vi "Can Connect Channels.vi"(8 "error in (no error)":errorcluster, 9 "channel 2":string, 10 "channel 1":string, 11 "session in":T2) -> (0 "error out":errorcluster, 2 "path capability":T1=1 items=["Path Available"=1, "Path Exists"=2, "Path Unsupported"=3, "Resource in Use"=4, "Source Conflict"=5, "Channel Not Available"=6], 3 "session out":T2)   [LabVIEW 2020, in "SLSC Switch.lvlib"]
doc: "Verifies that a path between <B>channel 1</B> and <B>channel 2</B> can be created.\n\nIf a path is possible in the switch module, the availability of that path is returned given the existing connections. If the path is possible but in use, an Implicit Connection Exists warning is returned."
uses:
  <vilib>/SLSC_Switch/SLSC Switch.lvlib
  nislscsl.dll
  <vilib>/userdefined/High Color/SLSC_Switch/nislscslSession.ctl
  <vilib>/SLSC_Switch/Path Capability.ctl
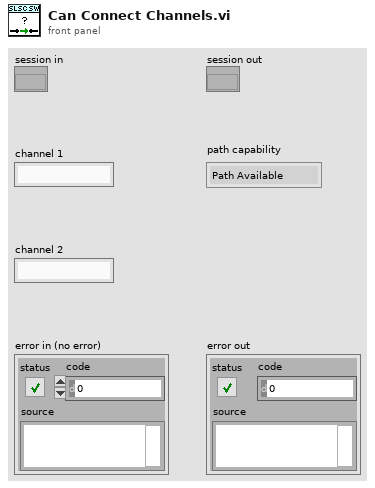
[diagram p1: front panel]
types:
  T1 = typedef "SLSC Switch.lvlib/Path Capability.ctl" = i32
  T2 = typedef "nislscslSession.ctl" = refnum<k20>
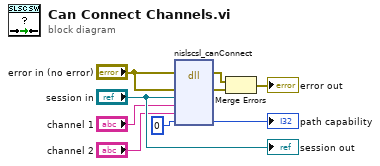
[diagram p0: block diagram]
diagram:
  n1 = dll-call lib="nislscsl.*" fn="nislscsl_canConnect"(error in="error in (no error)", "errorCluster"="error in (no error)", "sessionHandle"="session in", "channel 1"="channel 1", "channel 2"="channel 2", "path capability"=0) -> (error out=w8:errorcluster, "errorCluster"=w7:errorcluster, "path capability"=→"path capability":i32)  [unwired: 6 in, 1 out]
  n2 = Merge Errors(w8, w7) -> (→"error out":errorcluster)
  "session out" <- "session in"
